vi "Prioridade_variaveis_client.vi"() -> ()   [LabVIEW 2019]
uses:
  <vilib>/Utility/config.llb/Config Data RefNum.ctl
  padrao_TAGS_prioridades_client.ctl
  <vilib>/Utility/config.llb/Read Key (Boolean).vi
  <vilib>/Utility/config.llb/Write Key (Boolean).vi
  <vilib>/Utility/config.llb/NI_LVConfig.lvlib
panel:
  in  "Search Button":bool
  in  "BARRA DE PESQUISA":string
  out "padrao_prioridade_TAGs_nao_modificado":T1
  in  "padrao_prioridade_TAGs":T1
  in  "Cancelar Modificacao":bool
  in  "[ESC]":bool
  in  "Salvar":bool
  out "Status":string
  out "refnum out":T2
  out "error out":errorcluster
  # "SELECIONE AS VARIÁVEIS QUE ESSA APLICAÇÃO TEM PRIORIDADE"
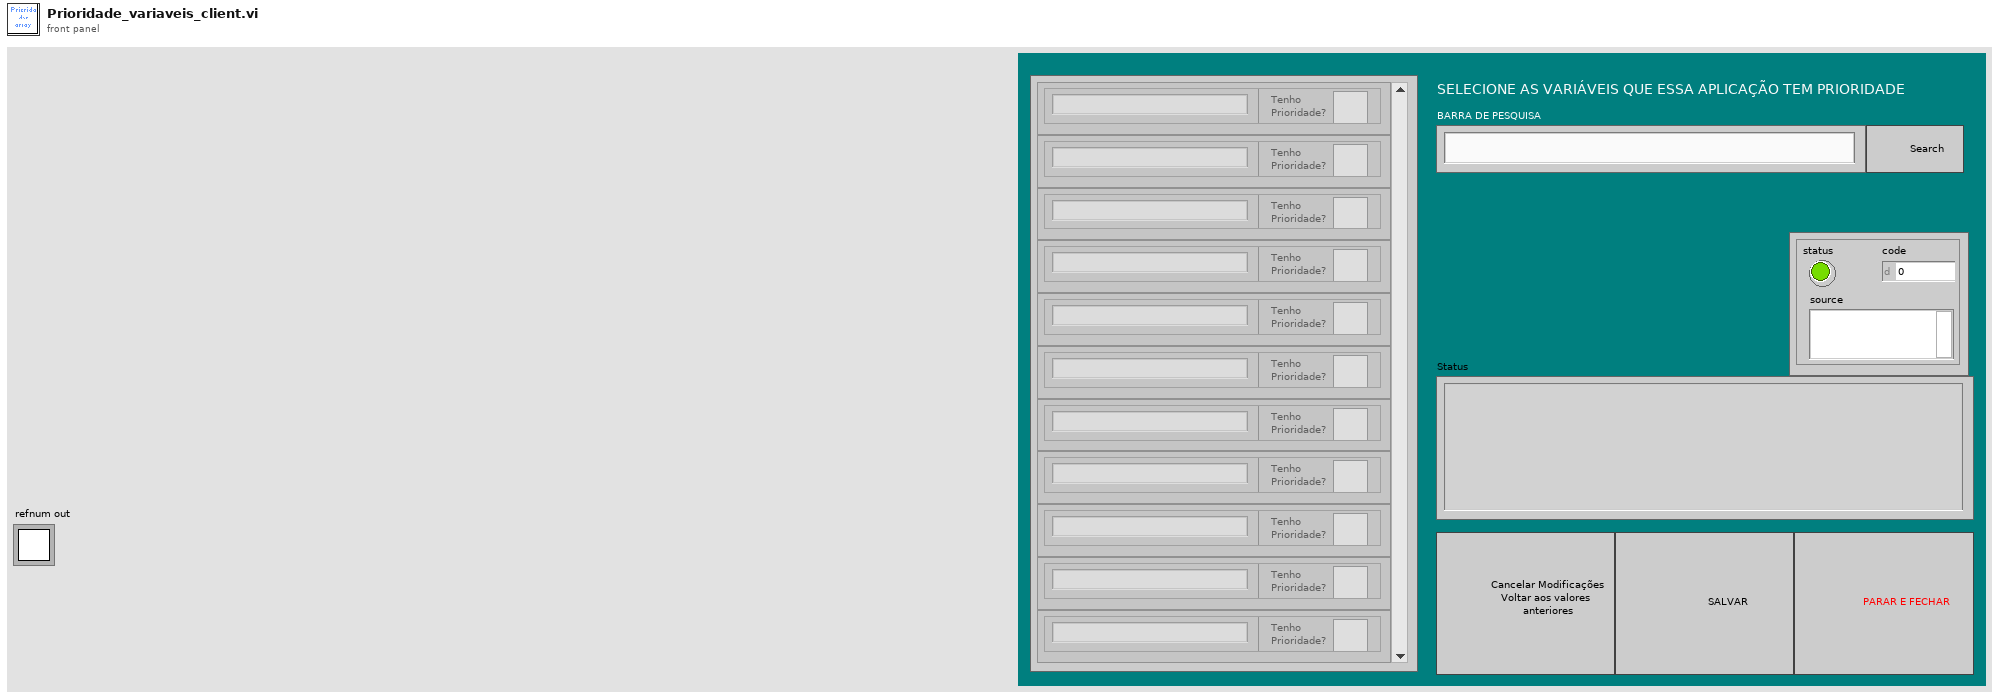
[diagram p1: front panel]
types:
  T1 = typedef "padrao_TAGS_prioridades_client.ctl" = cluster{"TAG":string, "Tenho\nPrioridade?":bool}[]
  T2 = typedef "NI_LVConfig.lvlib/Config Data RefNum.ctl" = refnum<k1>
  T3 = enum8{"Enabled", "Disabled", "Disabled and Grayed Out"}
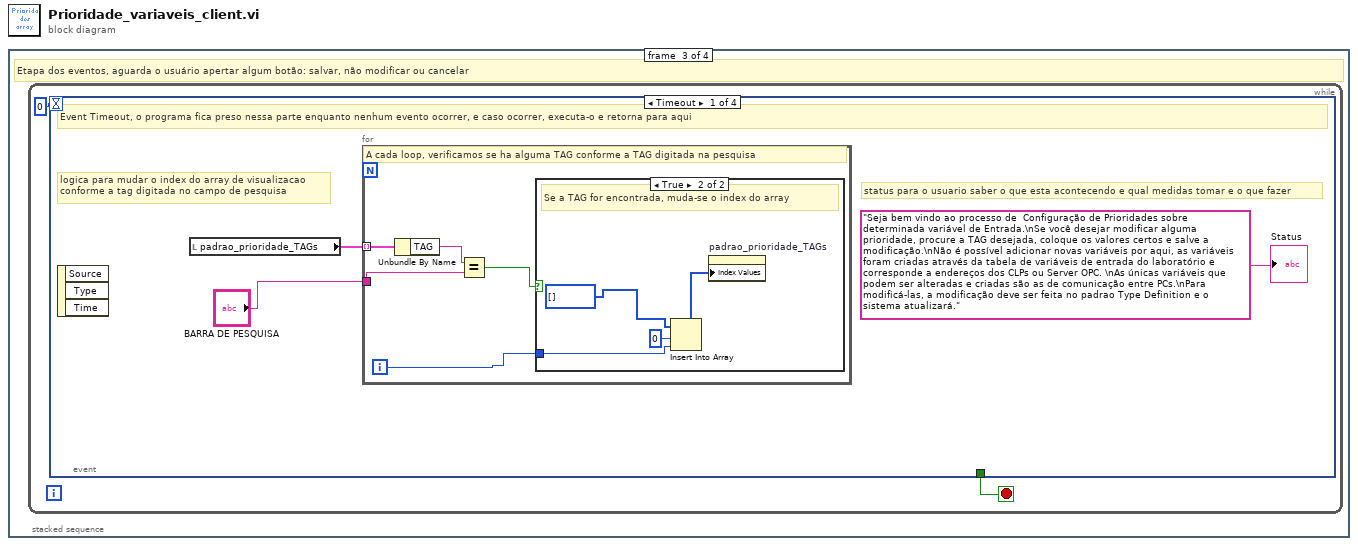
[diagram p0: block diagram]
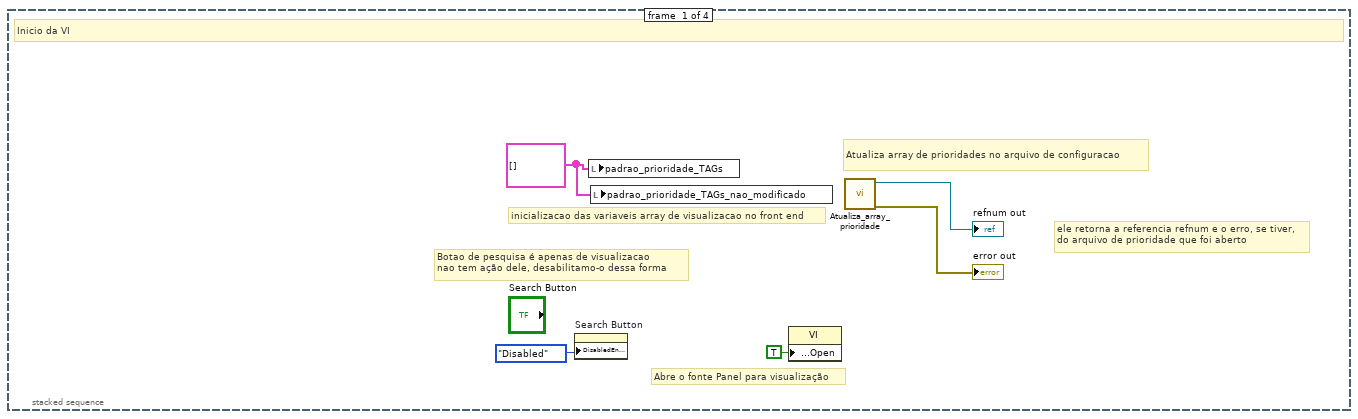
[diagram p2: hidden frame]
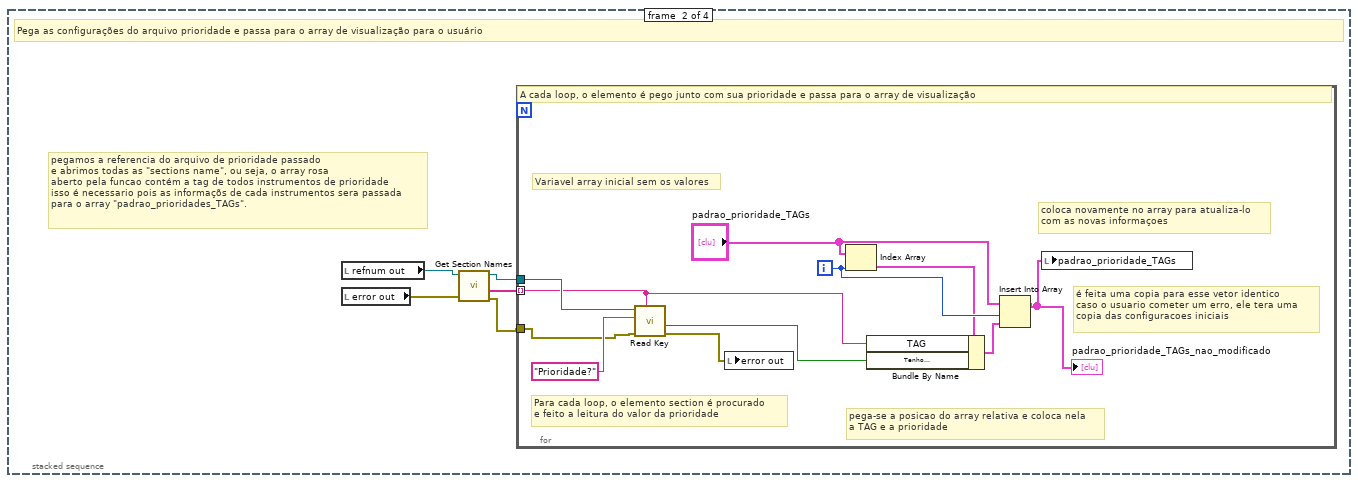
[diagram p3: hidden frame]
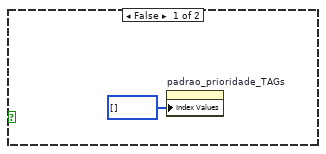
[diagram p4: hidden frame]
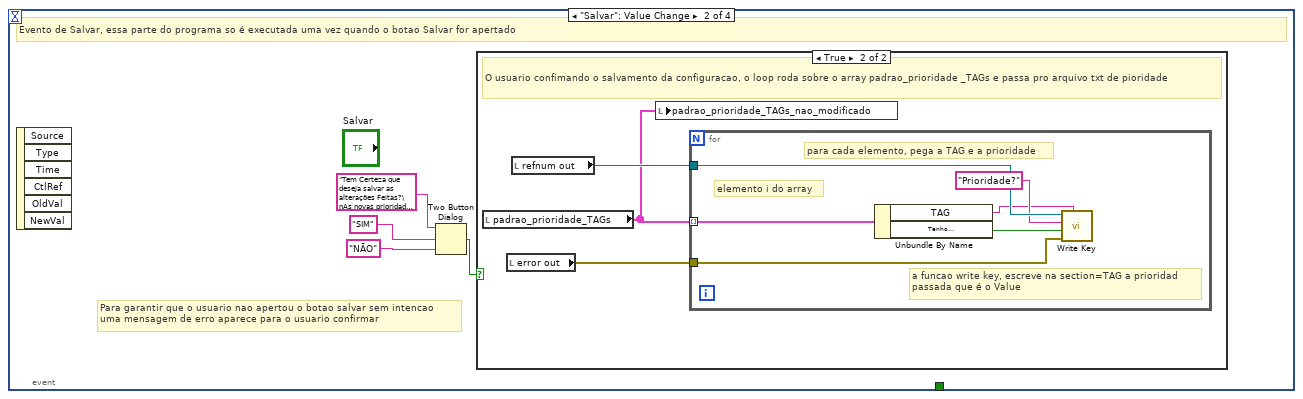
[diagram p5: hidden frame]
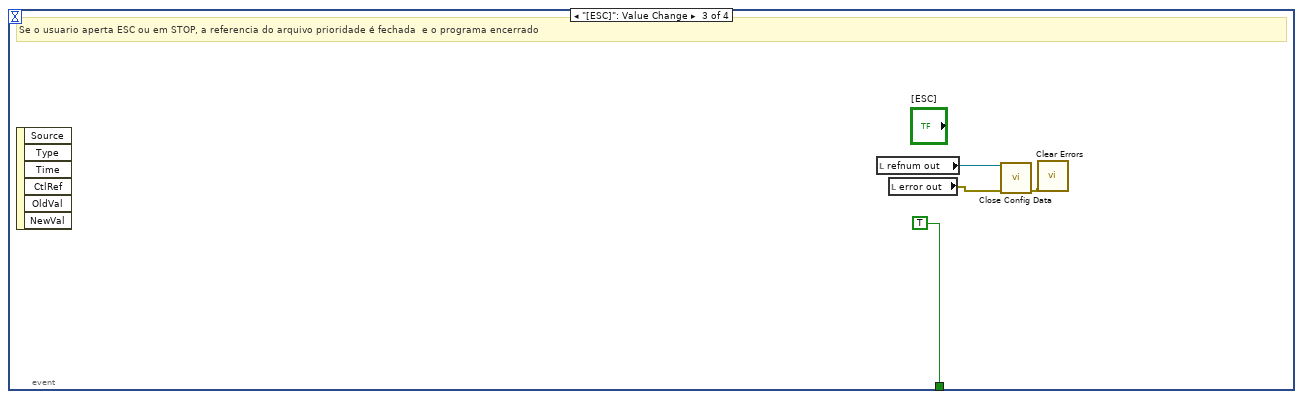
[diagram p7: hidden frame]
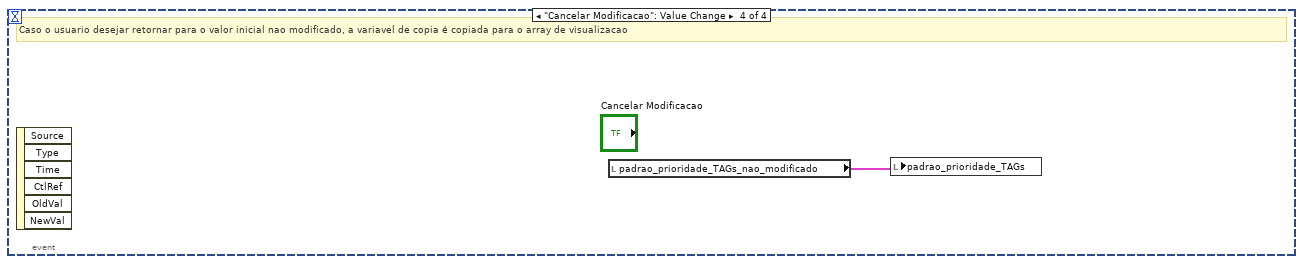
[diagram p8: hidden frame]
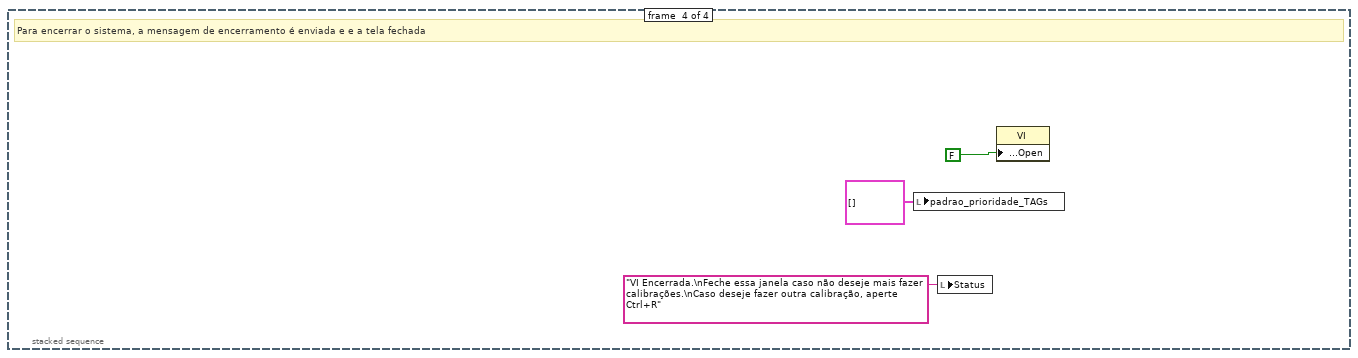
[diagram p9: hidden frame]
diagram:
  n1 = stacked-sequence {
    frame #0 {
      w4 = T1 [] ("padrao_prioridade_TAGs")
      # "ele retorna a referencia refnum e o erro, se tiver,\ndo arquivo de prioridade que foi aberto"
      # "inicializacao das variaveis array de visualizacao no front end"
      # "Botao de pesquisa é apenas de visualizacao\nnao tem ação dele, desabilitamo-o dessa forma"
      # "Abre o fonte Panel para visualização"
      # "Atualiza array de prioridades no arquivo de configuracao"
      # "Inicio da VI"
      n2 = property on="Search Button" class="Bool"("DisabledEnum"=T3."Disabled" ("Disabled")) -> ()  [unwired: 2 in, 2 out]
      n3 = local write "padrao_prioridade_TAGs"(w4) -> ()
      n4 = local write "padrao_prioridade_TAGs_nao_modificado"(w4) -> ()
      n5 = property class="VI"("Front Panel.Open"=TRUE ("Front Panel Window:Open")) -> ()  [unwired: 2 in, 2 out]
      n6 = call "Atualiza_array_prioridade.vi"() -> ("error out"=→"error out":errorcluster, "refnum"=→"refnum out":T2)  [unwired: 10 in]
    }
    frame #1 {
      # "pegamos a referencia do arquivo de prioridade passado\ne abrimos todas as \"sections name\", ou seja, o array rosa\naberto pela funcao contém a tag de todos instrumentos de prioridade\nisso é necessario pois as informaçõs de cada instrumentos sera passada\npara o array \"padrao_prioridades_TAGs\"."
      # "Pega as configurações do arquivo prioridade e passa para o array de visualização para o usuário"
      n7 = local read "refnum out"() -> (w10:T2)
      n8 = local read "error out"() -> (w7:errorcluster)
      n9 = call <vilib>:"Get Section Names.vi"("error in (no error)"=w7, "refnum"=w10) -> ("error out"=w6:errorcluster, "section names"=w9:string[], "refnum out"=w8:T2)  [unwired: 7 in]
      n10 = for {
        tunnel: w9 -> [w16] mode=indexing
        tunnel: w8 -> [w21]
        tunnel: w6 -> [w14]
        i -> [w19]
        # "é feita uma copia para esse vetor identico\ncaso o usuario cometer um erro, ele tera uma \ncopia das configuracoes iniciais"
        # "coloca novamente no array para atualiza-lo\ncom as novas informaçoes"
        # "pega-se a posicao do array relativa e coloca nela\na TAG e a prioridade"
        # "Para cada loop, o elemento section é procurado\ne feito a leitura do valor da prioridade"
        # "Variavel array inicial sem os valores"
        # "A cada loop, o elemento é pego junto com sua prioridade e passa para o array de visualização"
        n11 = call-poly <vilib>:"Read Key.vi"("section"=w16, "error in (no error)"=w14, "key"="Prioridade?", "refnum"=w21) -> ("error out"=w13:errorcluster, "value"=w15:bool)  [unwired: 4 in, 2 out]
        n12 = local write "error out"(w13) -> ()
        n13 = Index Array(array="padrao_prioridade_TAGs", index=w19) -> (element=w18:cluster{"TAG":string, "Tenho\nPrioridade?":bool})
        n14 = Bundle By Name(cluster=w18, "TAG"=w16, "Tenho\nPrioridade?"=w15) -> (w17:cluster{"TAG":string, "Tenho\nPrioridade?":bool})
        n15 = Insert Into Array(array="padrao_prioridade_TAGs", index=w19, new element=w17) -> (w11:T1)
        "padrao_prioridade_TAGs_nao_modificado" <- w11
        n16 = local write "padrao_prioridade_TAGs"(w11) -> ()
      }
    }
    frame #2 {
      # "Etapa dos eventos, aguarda o usuário apertar algum botão: salvar, não modificar ou cancelar"
      n17 = while {
        stop <- w23 stop-if-true
        n18 = event shown="[0] Timeout" {
          selector: _ -> [_ _ _ _]
          dyn-events: _ -> [_ _ _ _]
          timeout: 0 -> [_ _ _ _]
          tunnel: [_ _ TRUE _] -> w23
          event Timeout {
            # "logica para mudar o index do array de visualizacao \nconforme a tag digitada no campo de pesquisa"
            # "status para o usuario saber o que esta acontecendo e qual medidas tomar e o que fazer"
            # "Event Timeout, o programa fica preso nessa parte enquanto nenhum evento ocorrer, e caso ocorrer, executa-o e retorna para aqui"
            n19 = event-data() -> ()  [unwired: 1 in, 3 out]
            n20 = local read "padrao_prioridade_TAGs"() -> (w25:T1)
            n21 = for {
              tunnel: w25 -> [w31] mode=indexing
              tunnel: "BARRA DE PESQUISA" -> [w29]
              i -> [w28]
              # "A cada loop, verificamos se ha alguma TAG conforme a TAG digitada na pesquisa"
              n22 = Unbundle By Name(w31) -> ("TAG"=w30:string)
              n23 = Equal?(x=w30, y=w29) -> (x = y?=w27:bool)
              n24 = case shown="True" w27 {
                tunnel: w28 -> [_ w35]
                frame False {
                  n25 = property on="padrao_prioridade_TAGs" class="Arr (strict)"("Index Values"=u32[] []) -> ()  [unwired: 2 in, 2 out]
                }
                frame True {
                  # "Se a TAG for encontrada, muda-se o index do array"
                  n26 = Insert Into Array(array=u32[] [] ("Index Values"), index=0, new element=w35) -> (w33:u32[])
                  n27 = property on="padrao_prioridade_TAGs" class="Arr (strict)"("Index Values"=w33) -> ()  [unwired: 2 in, 2 out]
                }
              }
            }
            "Status" <- "Seja bem vindo ao processo de  Configuração de Prioridades sobre determinada variável de Entrada.\nSe você desejar modificar alguma prioridade, procure a TAG desejada, coloque os valores certos e salve a modificação.\nNão é possível adicionar novas variáveis por aqui, as variáveis foram criadas através da tabela de variáveis de entrada do laboratório e corresponde a endereços dos CLPs ou Server OPC. \nAs únicas variáveis que podem ser alteradas e criadas são as de comunicação entre PCs.\nPara modificá-las, a modificação deve ser feita no padrao Type Definition e o sistema atualizará." ("Status")
          }
          event "Salvar": Value Change {
            # "Para garantir que o usuario nao apertou o botao salvar sem intencao\numa mensagem de erro aparece para o usuario confirmar"
            # "Evento de Salvar, essa parte do programa so é executada uma vez quando o botao Salvar for apertado"
            n28 = event-data() -> ()  [unwired: 1 in, 6 out]
            n29 = Two Button Dialog(message="Tem Certeza que deseja salvar as alterações Feitas?\nAs novas prioridades serão estabelecidas e a antiga configuração será perdida", 1:"NÃO" ("F button name (\"Cancel\")"), 2:"SIM" ("T button name (\"OK\")")) -> (T button?=w40:bool)
            n30 = case shown="True" w40 {
              frame False {
                # "Caso ele cancelar o salvamento, nada acontece e volta para a tela de timeout para o usuario escolher o que fazer"
              }
              frame True {
                # "O usuario confimando o salvamento da configuracao, o loop roda sobre o array padrao_prioridade _TAGs e passa pro arquivo txt de pioridade"
                n31 = local read "padrao_prioridade_TAGs"() -> (w41:T1)
                n32 = local read "error out"() -> (w42:errorcluster)
                n33 = local read "refnum out"() -> (w43:T2)
                n34 = local write "padrao_prioridade_TAGs_nao_modificado"(w41) -> ()
                n35 = for {
                  tunnel: w43 -> [w48]
                  tunnel: w42 -> [w49]
                  tunnel: w41 -> [w46] mode=indexing
                  # "a funcao write key, escreve na section=TAG a prioridad\npassada que é o Value"
                  # "para cada elemento, pega a TAG e a prioridade"
                  # "elemento i do array"
                  n36 = Unbundle By Name(w46) -> ("TAG"=w45:string, "Tenho\nPrioridade?"=w44:bool)
                  n37 = call-poly <vilib>:"Write Key.vi"("section"=w45, "error in (no error)"=w49, "value"=w44, "key"="Prioridade?", "refnum"=w48) -> ()  [unwired: 4 in, 3 out]
                }
              }
            }
          }
          event "[ESC]": Value Change {
            # "Se o usuario aperta ESC ou em STOP, a referencia do arquivo prioridade é fechada  e o programa encerrado"
            n38 = event-data() -> ()  [unwired: 1 in, 6 out]
            n39 = local read "refnum out"() -> (w52:T2)
            n40 = local read "error out"() -> (w50:errorcluster)
            n41 = call <vilib>:"Close Config Data.vi"("error in (no error)"=w50, "refnum"=w52) -> ("error out"=w51:errorcluster)  [unwired: 8 in, 1 out]
            n42 = call <vilib>:"Clear Errors.vi"("error in (no error)"=w51) -> ()  [unwired: 5 in, 2 out]
          }
          event "Cancelar Modificacao": Value Change {
            # "Caso o usuario desejar retornar para o valor inicial nao modificado, a variavel de copia é copiada para o array de visualizacao"
            n43 = event-data() -> ()  [unwired: 1 in, 6 out]
            n44 = local read "padrao_prioridade_TAGs_nao_modificado"() -> (w54:T1)
            n45 = local write "padrao_prioridade_TAGs"(w54) -> ()
          }
        }
      }
    }
    frame #3 {
      # "Para encerrar o sistema, a mensagem de encerramento é enviada e e a tela fechada"
      n46 = local write "padrao_prioridade_TAGs"(T1 [] ("padrao_prioridade_TAGs")) -> ()
      n47 = local write "Status"("VI Encerrada.\nFeche essa janela caso não deseje mais fazer calibrações.\nCaso deseje fazer outra calibração, aperte Ctrl+R" ("Status")) -> ()
      n48 = property class="VI"("Front Panel.Open"=FALSE ("Front Panel Window:Open")) -> ()  [unwired: 2 in, 2 out]
    }
  }
